vi "solar_write VoyagerPacketsOverride.vi"(8 "error in (no error)":errorcluster, 10 "PACKETS":T1[](array[typedef]) {"last_time" format="%<%H:%M:%S%3u %m/%d/%y>T"}, 11 "solar in":refnum<class "solar.lvclass">) -> (0 "error out":errorcluster, 3 "solar out":refnum<class "solar.lvclass">)   [LabVIEW 2018, in "solar.lvclass"]
doc: "This registers Voyager packet definitions for the Voyager interface <b>and overrides the packet if it already exists.</b> When a Voyager target is registered, the COSMOS command & telemetry definitions are automatically loaded. \n- Each packet must specifiy CMD|TLM, TARGET & PACKET names. \n - If the ID field is 0, Voyager assigns a new available ID. \n - Each packet item must contain the item NAME, SIZE, TYPE and LVTYPE as a minimum. \n - Use the Voyager Definition Import VIs to generate the Packets from a control refnum, variant, etc.\n<b>If the packet is already registered, this overrides the existing packet</b>"
uses:
  solar.lvclass
  voyager/solar_voy_def/solar_voy_def_ctl ITEM.ctl
  voyager/solar_voy_def/solar_voy_def_ctl PACKET.ctl
  voyager/solar_voy_def/solar_voy_def_ctl ITEM TYPE.ctl
  type/solar_type Item Type.ctl
  voyager/solar_voy_def/solar_voy_def_ctl PACKET_ID.ctl
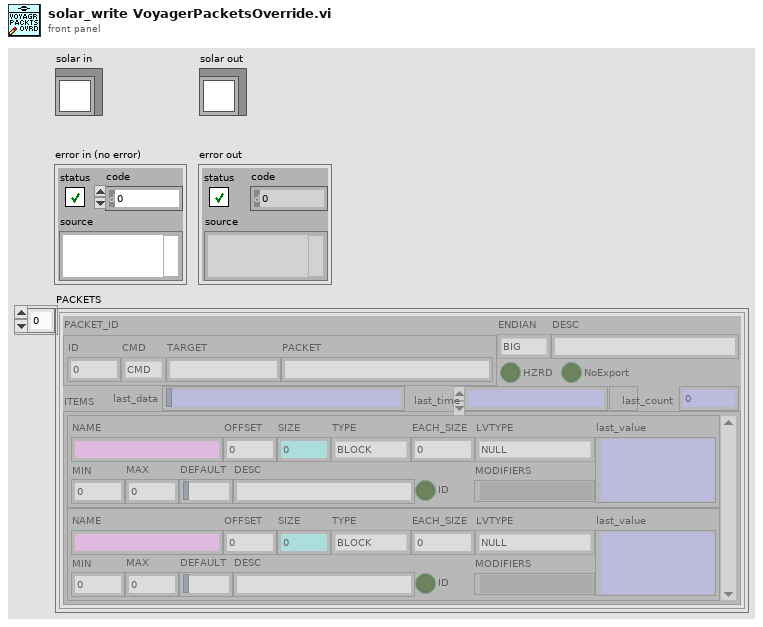
[diagram p1: front panel]
types:
  T1 = typedef "solar_voy_def_ctl PACKET.ctl" = cluster{"PACKET_ID":T2, "ENDIAN":enum8{"BIG", "LITTLE"}, "DESC":string, "HZRD":bool, "ITEMS":T3[], "NoExport":bool, "last_time":timestamp, "last_count":u32, "last_data":string}
  T2 = typedef "solar_voy_def_ctl PACKET_ID.ctl" = cluster{"ID":u16, "CMD":enum8{"CMD", "TLM"}, "TARGET":string, "PACKET":string}
  T3 = typedef "solar_voy_def_ctl ITEM.ctl" = cluster{"NAME":string, "OFFSET":i32, "SIZE":i32, "TYPE":T4, "EACH_SIZE":i32, "LVTYPE":T5, "MIN":dbl, "MAX":dbl, "DEFAULT":string, "DESC":string, "ID":bool, "MODIFIERS":variant, "last_value":variant}
  T4 = typedef "solar_voy_def_ctl ITEM TYPE.ctl" = enum8{"BLOCK", "INT", "UINT", "FLOAT", "STRING"}
  T5 = typedef "solar_type Item Type.ctl" = enum16{"NULL", "UNKNOWN", "CLUSTER", "I8", "I16", "I32", "I64", "U8", "U16", "U32", "U64", "U8_ENUM", "U16_ENUM", "U32_ENUM", "SGL", "DBL", "BOOLEAN", "STRING", "PATH", "VISA", "TAG", "TIME", "I8_1D", "I16_1D", "I32_1D", "I64_1D", "U8_1D", "U16_1D", "U32_1D", "U64_1D", "U8_ENUM_1D", "U16_ENUM_1D", "U32_ENUM_1D", "SGL_1D", "DBL_1D", "BOOLEAN_1D", "STRING_1D", "PATH_1D", "VISA_1D", "TAG_1D", "TIME_1D", "I8_2D", "I16_2D", "I32_2D", "I64_2D", "U8_2D", "U16_2D", "U32_2D", "U64_2D", "U8_ENUM_2D", "U16_ENUM_2D", "U32_ENUM_2D", "SGL_2D", "DBL_2D", "BOOLEAN_2D", "STRING_2D", "PATH_2D", "VISA_2D", "TAG_2D", "TIME_2D"}
  T6 = typedef "solar_ctl SOLAR Refnum.ctl" = refnum<k1>
  T7 = typedef "solar_ctl SOLAR Global.ctl" = cluster{"Targets":T8[], "AppDir":path, "solar.ini":path, "ConfigsDir":path, "CosmosDir":path, "LogsDir":path, "ExePath":path, "ExeVersion":string, "PartNum":string, "AppSetup":string, "Title":string, "Main.ini":path, "Temp.ini":path, "vSOLAR":string, "Splash.png":string, "SplashWait":i32, "SOLARUE":refnum<user-event>, "VoyagerRefnum":T9, "QTimerRefnum":T10}
  T8 = typedef "solar_ctl Target Global.ctl" = cluster{"Target":string, "Q":refnum<queue>, "UE":refnum<user-event>, "VI":refnum<vi>, "Menu":refnum<k9>, "Data":refnum<data-value>, "Attributes":variant}
  T9 = typedef "solar_voy_ctl Voyager Refnum.ctl" = refnum<k1>
  T10 = typedef "solar_qtimer_ctl Refnum.ctl" = refnum<k1>
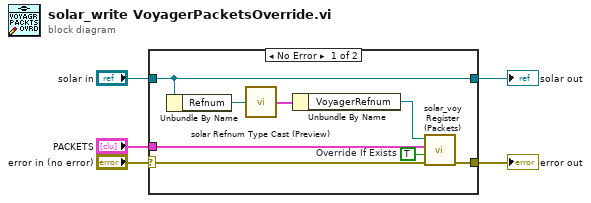
[diagram p0: block diagram]
diagram:
  n1 = case shown="No Error" "error in (no error)" {
    selector: "error in (no error)" -> [w11 w15]
    tunnel: "solar in" -> [w7 w14]
    tunnel: [w10 w15] -> w3
    tunnel: "PACKETS" -> [w9 _]
    tunnel: [w7 w14] -> w1
    frame No Error {
      w6 = TRUE  # Override If Exists
      n2 = Unbundle By Name(w7) -> ("Refnum"=w12:T6)
      n3 = call "solar Refnum Type Cast (Preview).vi"("Refnum"=w12) -> ("SOLAR"=w13:T7)  [unwired: 8 in]
      n4 = Unbundle By Name(w13) -> ("VoyagerRefnum"=w8:T9)
      n5 = call "solar_voy Register (Packets).vi"("error in (no error)"=w11, "Override If Exists? (F)"=w6, "PACKETS (No HDR)"=w9, "Voyager Refnum in"=w8) -> ("error out"=w10:errorcluster)  [unwired: 6 in, 1 out]
    }
    frame Error {
    }
  }
  "error out" <- w3
  "solar out" <- w1
